vi "GoTo Tangent.vi"(7 "IA State Input in":T2, 8 "distance between ball and robot":dbl=250.0 format="%#_13g", 9 "Ball":dbl[](array[numeric])=[-1986.6092529296875, -3009.6396484375], 10 "Target":dbl[](array[numeric]), 11 "R":dbl[](array[numeric])=[-2840.578369140625, -1536.7857666015625, -1.0371381044387817]) -> (1 "Destination":dbl[](array[numeric]), 2 "Output\nVelocity":dbl[](array[numeric]) format="%.2f")   [LabVIEW 2016]
uses:
  Core/AI Input.ctl
  Core/AI Robot.ctl
  Intel/Functions Enum.ctl
  Intel/AttackerStates.ctl
  Core/AI Ball.ctl
  Core/Field Size.ctl
  Core/AI Judge.ctl
  Intel/Command Enum.ctl
  Util/Events/Events.ctl
  <vilib>/Analysis/coordinate.llb/Angle Range (Degree).ctl
  <vilib>/Analysis/coordinate.llb/Wrap Angle (scalar).vi
  <vilib>/Analysis/coordinate.llb/2D Cartesian Coordinate Rotation (Scalar).vi
  <vilib>/Analysis/NI_AALPro.lvlib
  <vilib>/Analysis/NI_AAL_Angle.lvlib
panel:
  in  "angle range":T1=1 items=["none", "-180 to 180 (-pi to pi)", "0 to 360 (0 to 2pi)"]
  out "Waveform Chart 2":dbl[][](graph)
  out "Robot":dbl[](array[numeric])=[-2840.578369140625, -1536.7857666015625, -1.0371381044387817]
  out "Waveform Chart":dbl[][](graph)
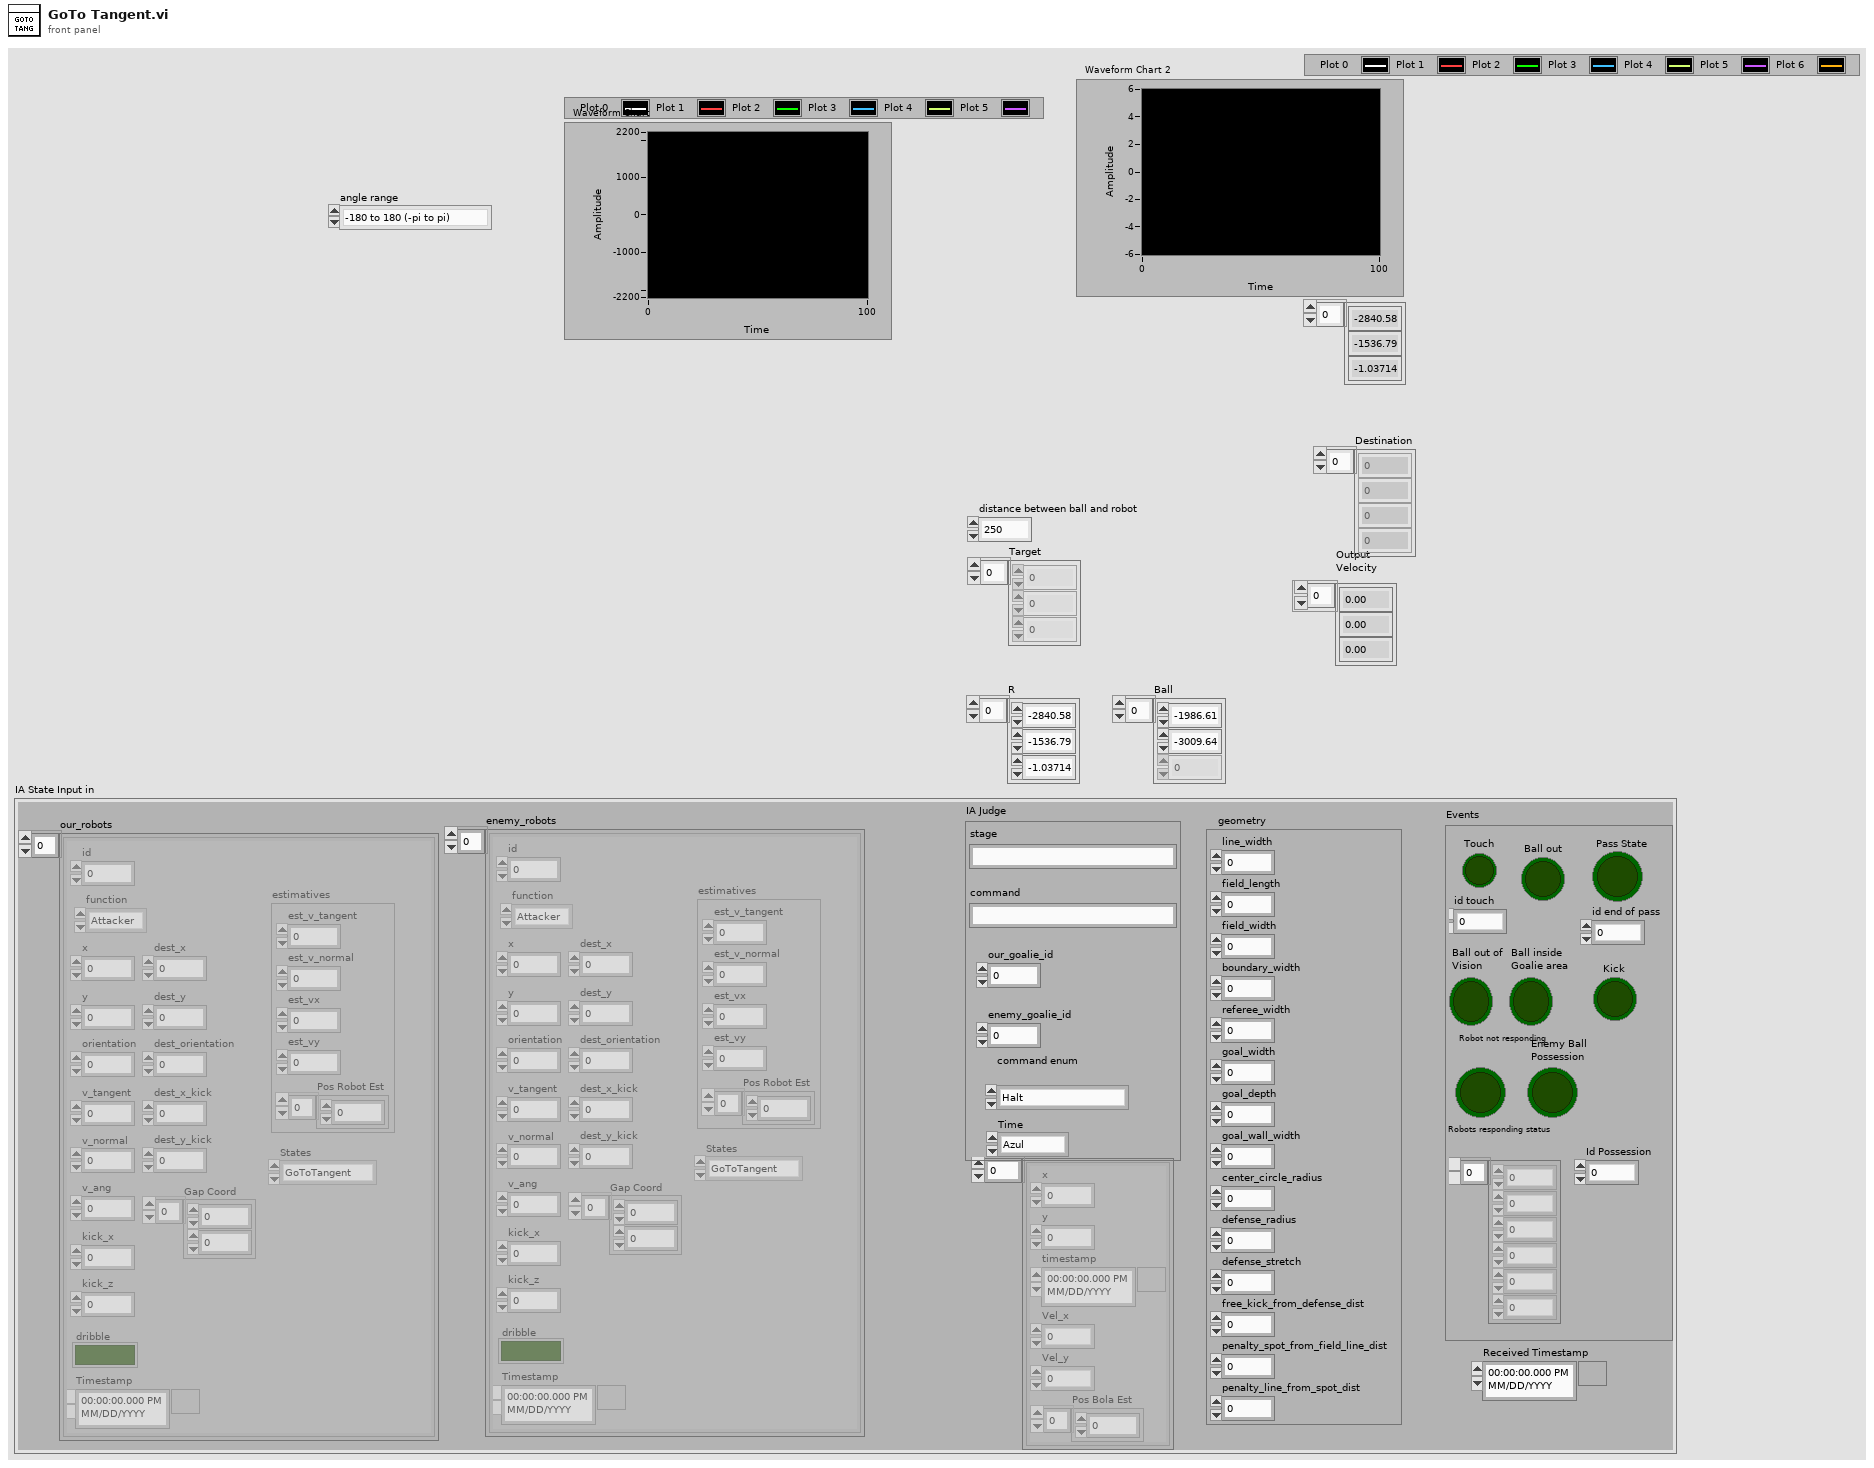
[diagram p1: front panel]
types:
  T1 = typedef "NI_AAL_Angle.lvlib/Angle Range (Degree).ctl" = u16
  T2 = typedef "AI Input.ctl" = cluster{"our_robots":T3[], "enemy_robots":T3[], "balls":T6[], "geometry":T7, "IA Judge":T8, "Received Timestamp":timestamp, "Events":T10}
  T3 = typedef "AI Robot.ctl" = cluster{"id":u32, "function":T4, "x":dbl, "y":dbl, "orientation":dbl, "v_tangent":dbl, "v_normal":dbl, "v_ang":dbl, "kick_x":dbl, "kick_z":dbl, "dribble":bool, "Timestamp":timestamp, "dest_x":dbl, "dest_y":dbl, "dest_orientation":dbl, "estimatives":cluster{"est_v_tangent":dbl, "est_v_normal":dbl, "est_vx":dbl, "est_vy":dbl, "Pos Robot Est":dbl[]}, "dest_x_kick":dbl, "dest_y_kick":dbl, "Gap Coord":dbl[], "States":T5}
  T4 = typedef "Functions Enum.ctl" = enum16{"Attacker", "Goalie", "Defender", "Striker", "Goto 0", "Dummy", "Kicker", "ZigZag"}
  T5 = typedef "AttackerStates.ctl" = enum16{"Pass", "GoToTangent", "BallGetting", "GoToKick", ""}
  T6 = typedef "AI Ball.ctl" = cluster{"x":dbl, "y":dbl, "timestamp":timestamp, "Vel_x":dbl, "Vel_y":dbl, "Pos Bola Est":dbl[]}
  T7 = typedef "Field Size.ctl" = cluster{"line_width":u32, "field_length":u32, "field_width":u32, "boundary_width":u32, "referee_width":u32, "goal_width":u32, "goal_depth":u32, "goal_wall_width":u32, "center_circle_radius":u32, "defense_radius":u32, "defense_stretch":u32, "free_kick_from_defense_dist":u32, "penalty_spot_from_field_line_dist":u32, "penalty_line_from_spot_dist":u32}
  T8 = typedef "AI Judge.ctl" = cluster{"stage":string, "command":string, "our_goalie_id":dbl, "enemy_goalie_id":dbl, "command enum":T9, "Time":enum16{"Azul", "Amarelo"}}
  T9 = typedef "Command Enum.ctl" = enum16{"Halt", "Stop", "Force Start", "PKA Normal Start", "Prepare Kickoff Ally", "PKE Normal Start", "Prepare Kickoff Enemy", "Prepare Penalty Ally", "PPA Normal Start", "Prepare Penalty Enemy", "PPE Normal Start", "Direct Free Enemy", "Direct Free Ally", "Indirect Free Enemy", "Indirect Free Ally", "Timeout Enemy", "Timeout Ally", "Goal Enemy", "Goal Ally", "Ball Placement Enemy", "Ball Placement Ally", "Normal Half Time", "Extra Time Break", "Extra Half Time", "None"}
  T10 = typedef "Events.ctl" = cluster{"Touch":bool, "Ball out":bool, "id touch":dbl, "Ball out of \nVision":bool, "Ball inside \nGoalie area":bool, "Robot not responding":bool, "Robots responding status":dbl[], "Enemy Ball \nPossession":bool, "Pass State":bool, "id end of pass":dbl, "Kick":bool, "Id Possession":dbl}
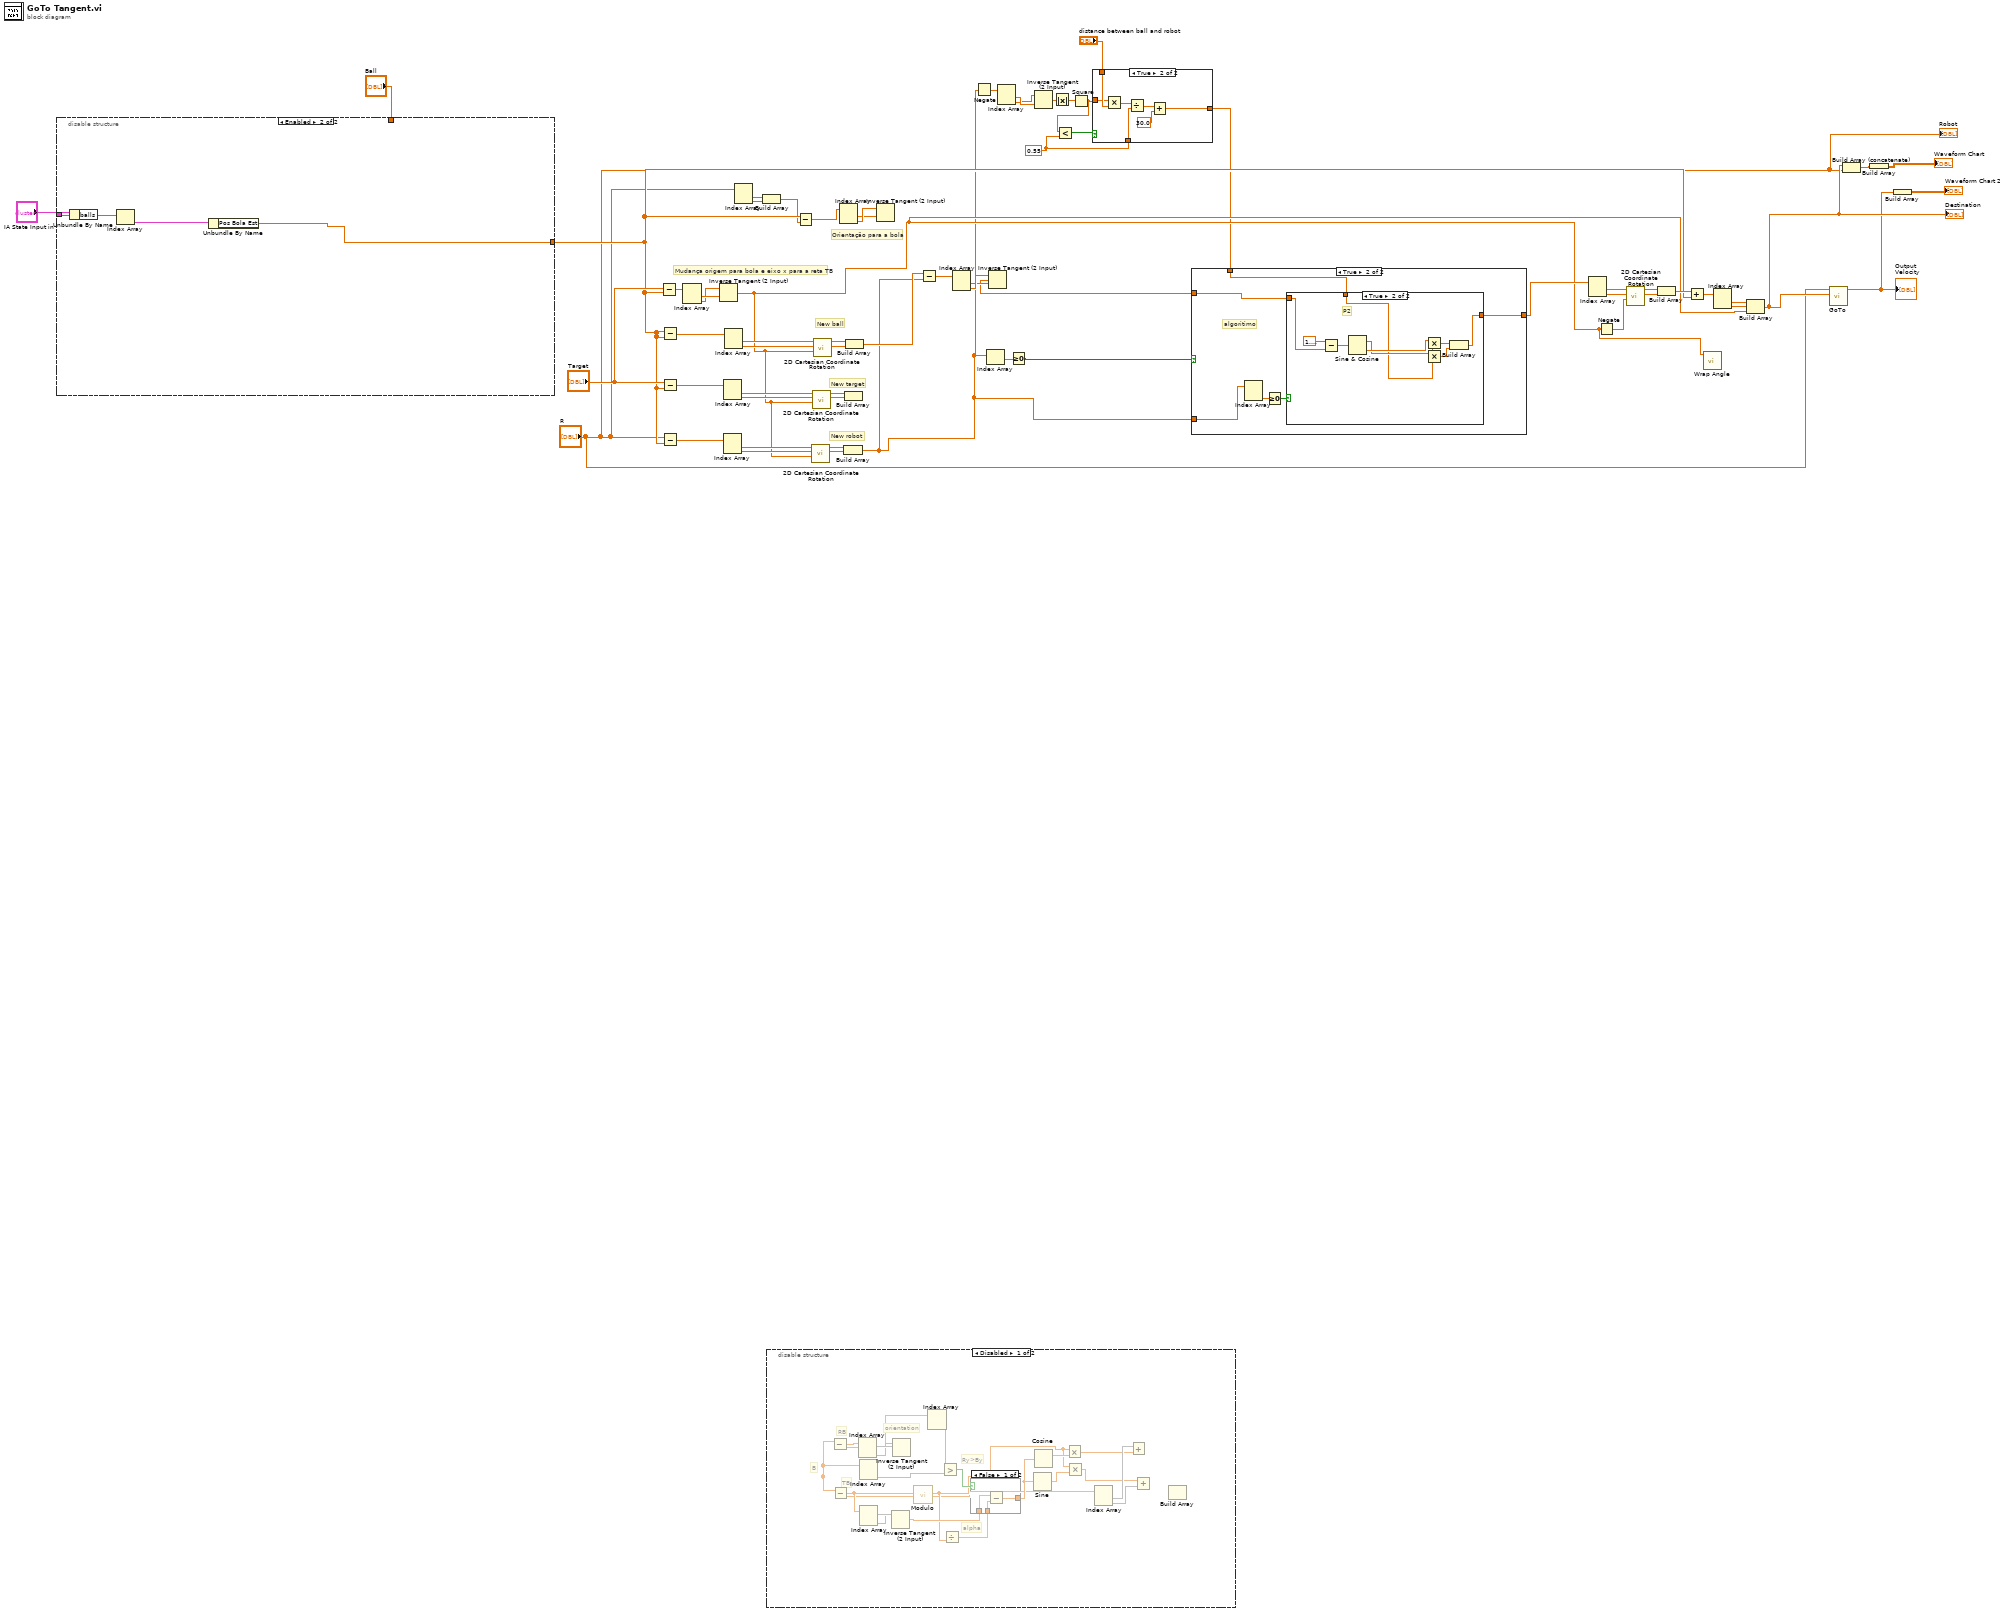
[diagram p0: block diagram]
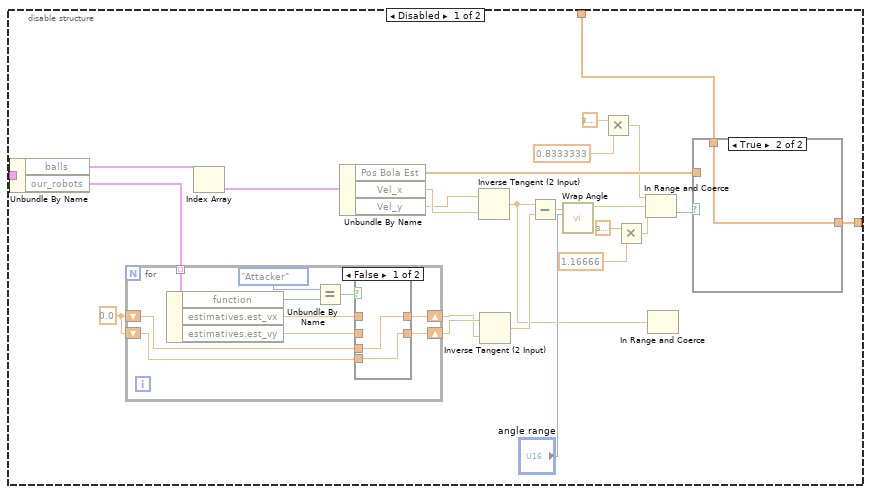
[diagram p3: hidden frame]
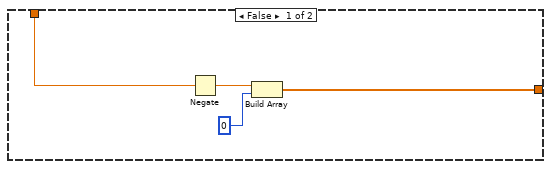
[diagram p6: hidden frame]
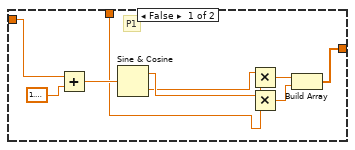
[diagram p7: hidden frame]
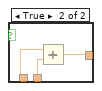
[diagram p8: hidden frame]
diagram:
  w5 = 0.55 ("y")
  # "New ball"
  # "New target"
  # "New robot"
  # "Orientação para a bola"
  # "Mudança origem para bola e eixo x para a reta TB"
  n1 = disable-structure shown="Enabled" {
    disable-tunnel: [w87 w103] -> w19
    disable-tunnel: "IA State Input in" -> [w86 w106]
    disable-tunnel: "Ball" -> [w64 _]
    frame Disabled {
      w82 = 0.0 ("est_vx")
      n2 = Unbundle By Name(w86) -> ("balls"=w85:T6[], "our_robots"=w83:T3[])
      n3 = for {
        tunnel: w83 -> [w97] mode=indexing
        shift-right: [w93] -> w79
        shift-left: w82 -> [w89]
        shift-right: [w90] -> w80
        shift-left: w82 -> [w88]
        n4 = Unbundle By Name(w97) -> ("function"=w95:T4, "estimatives.est_vx"=w92:dbl, "estimatives.est_vy"=w91:dbl)
        n5 = Equal?(x=Functions_Enum."Attacker" ("function"), y=w95) -> (x = y?=w96:bool)
        n6 = case shown="False" w96 {
          tunnel: [w99 w101] -> w93
          tunnel: w92 -> [_ w101]
          tunnel: w91 -> [_ w100]
          tunnel: [w98 w100] -> w90
          tunnel: w89 -> [w99 _]
          tunnel: w88 -> [w98 _]
          frame False {
          }
          frame True {
          }
        }
      }
      n7 = Index Array(array=w85) -> (element=w84:T6)  [unwired: 1 in]
      n8 = Unbundle By Name(w84) -> ("Pos Bola Est"=w81:dbl[], "Vel_x"=w78:dbl, "Vel_y"=w77:dbl)
      n9 = Inverse Tangent (2 Input)(1:w78, 2:w77) -> (0:w65:dbl)
      n10 = Inverse Tangent (2 Input)(1:w79, 2:w80) -> (0:w76:dbl)
      n11 = Subtract(x=w65, y=w76) -> (x-y=w74:dbl)
      n12 = call-poly <vilib>:"Wrap Angle.vi"("angle range"="angle range", "angle in"=w74) -> ("angle out"=w70:dbl)  [unwired: 8 in, 1 out]
      n13 = Multiply(x=3.141592653589793, y=0.8333333) -> (x*y=w67:dbl)
      n14 = Multiply(x=3.141592653589793, y=1.16666) -> (x*y=w73:dbl)
      n15 = In Range and Coerce(upper limit=w67, x=w70, lower limit=w73) -> (In Range?=w66:bool)  [unwired: 1 out]
      n16 = In Range and Coerce(x=w65) -> ()  [unwired: 2 in, 2 out]
      n17 = case shown="True" w66 {
        tunnel: [_ w102] -> w87
        tunnel: w81 -> [_ _]
        tunnel: w64 -> [_ w102]
        frame False {
        }
        frame True {
        }
      }
    }
    frame Enabled {
      n18 = Unbundle By Name(w106) -> ("balls"=w104:T6[])
      n19 = Index Array(array=w104) -> (element=w105:T6)  [unwired: 1 in]
      n20 = Unbundle By Name(w105) -> ("Pos Bola Est"=w103:dbl[])
    }
  }
  n21 = Subtract(x="Target", y=w19) -> (x-y=w54:dbl[])
  n22 = Subtract(x=w19, y=w19) -> (x-y=w61:dbl[])
  n23 = Subtract(x="Target", y=w19) -> (x-y=w58:dbl[])
  n24 = Subtract(x="R", y=w19) -> (x-y=w55:dbl[])
  n25 = Index Array(array=w54) -> (element #1=w53:dbl, element #2=w52:dbl)  [unwired: 2 in]
  n26 = Inverse Tangent (2 Input)(1:w53, 2:w52) -> (0:w12:dbl)
  n27 = Index Array(array=w55) -> (element #1=w57:dbl, element #2=w56:dbl)  [unwired: 2 in]
  n28 = Index Array(array=w58) -> (element #1=w60:dbl, element #2=w59:dbl)  [unwired: 2 in]
  n29 = Index Array(array=w61) -> (element #1=w63:dbl, element #2=w62:dbl)  [unwired: 2 in]
  n30 = Index Array(array="R") -> (element #1=w17:dbl, element #2=w16:dbl)  [unwired: 2 in]
  n31 = Build Array(w17, w16) -> (w15:dbl[])
  n32 = disable-structure shown="Disabled" {
    frame Disabled {
      # "Ry>By"
      # "orientation"
      # "RB"
      # "alpha"
      # "TB"
      # "B"
      n33 = Index Array() -> (array=w112:dbl[], element #2=w118)  [unwired: 2 in, 1 out]
      n34 = Index Array() -> (array=w108:dbl[], element #2=w119)  [unwired: 2 in, 1 out]
      n35 = Subtract(x=w112, y=w108) -> (x-y=w126:dbl)
      n36 = Index Array(array=w126) -> (element #1=w128, element #2=w127)  [unwired: 2 in]
      n37 = Inverse Tangent (2 Input)(1:w128, 2:w127) -> (0:w125:dbl)
      n38 = Greater?(x=w119, y=w118) -> (0:w117:bool)
      n39 = Index Array() -> (array=w107:dbl[], element #1=w115, element #2=w110)  [unwired: 2 in]
      n40 = Subtract(x=w112, y=w107) -> (x-y=w130:dbl)
      n41 = Index Array(array=w130) -> (element #1=w132, element #2=w131)  [unwired: 2 in]
      n42 = Inverse Tangent (2 Input)(1:w132, 2:w131) -> (0:w124:dbl)
      n43 = call "Modulo.vi"("2D vector"=w130) -> ("Modulo"=w116:dbl)  [unwired: 10 in]
      n44 = Divide(y=w116) -> (x=w129:dbl, x/y=w123:dbl)
      n45 = case shown="False" w117 {
        tunnel: w124 -> [w134 w138]
        tunnel: w123 -> [w135 w137]
        tunnel: [w133 w136] -> w122
        frame False {
          n46 = Subtract(x=w134, y=w135) -> (x-y=w133:dbl)
        }
        frame True {
          n47 = Add(x=w138, y=w137) -> (x+y=w136:dbl)
        }
      }
      n48 = Sine(x=w122) -> (sin(x)=w120:dbl)
      n49 = Cosine(x=w122) -> (cos(x)=w121:dbl)
      n50 = Multiply(x=w116, y=w121) -> (x*y=w114:dbl)
      n51 = Multiply(x=w116, y=w120) -> (x*y=w111:dbl)
      n52 = Add(x=w115, y=w114) -> (x+y=w113:dbl)
      n53 = Add(x=w111, y=w110) -> (x+y=w109:dbl)
      n54 = Build Array() -> ()  [unwired: 3 in, 1 out]
    }
    frame Enabled {
    }
  }
  n55 = Subtract(x=w19, y=w15) -> (x-y=w34:dbl[])
  n56 = call-poly <vilib>:"2D Cartesian Coordinate Rotation.vi"("theta"=w12, "y"=w56, "x"=w57) -> ("y out"=w46:dbl, "x out"=w47:dbl)  [unwired: 6 in, 1 out]
  n57 = call-poly <vilib>:"2D Cartesian Coordinate Rotation.vi"("theta"=w12, "y"=w59, "x"=w60) -> ("y out"=w50:dbl, "x out"=w51:dbl)  [unwired: 6 in, 1 out]
  n58 = call-poly <vilib>:"2D Cartesian Coordinate Rotation.vi"("theta"=w12, "y"=w62, "x"=w63) -> ("y out"=w48:dbl, "x out"=w49:dbl)  [unwired: 6 in, 1 out]
  n59 = Index Array(array=w34) -> (element #1=w35:dbl, element #2=w36:dbl)  [unwired: 2 in]
  n60 = Build Array(w47, w46) -> (w11:dbl[])
  n61 = Build Array(w51, w50) -> ()  [unwired: 1 out]
  n62 = Build Array(w49, w48) -> (w27:dbl[])
  n63 = Inverse Tangent (2 Input)(1:w35, 2:w36) -> ()  [unwired: 1 out]
  n64 = Subtract(x=w27, y=w11) -> (x-y=w43:dbl[])
  n65 = Index Array(array=w43) -> (element #1=w44:dbl, element #2=w45:dbl)  [unwired: 2 in]
  n66 = Negate(x=w11) -> (-x=w10:dbl[])
  n67 = Index Array(array=w11) -> (element=w29:dbl)  [unwired: 1 in]
  n68 = Inverse Tangent (2 Input)(1:w44, 2:w45) -> (0:w28:dbl)
  n69 = Index Array(array=w10) -> (element #1=w9:dbl, element #2=w8:dbl)  [unwired: 2 in]
  n70 = Greater Or Equal To 0?(x=w29) -> (x >= 0?=w30:bool)
  n71 = Inverse Tangent (2 Input)(1:w9, 2:w8) -> (0:w7:dbl)
  n72 = Absolute Value(x=w7) -> (abs(x)=w2:dbl)
  n73 = Square(x=w2) -> (x^2=w1:dbl)
  n74 = Less?(x=w1, y=w5) -> (x < y?=w6:bool)
  n75 = case shown="True" w6 {
    tunnel: w5 -> [_ w143]
    tunnel: [w139 w142] -> w4
    tunnel: "distance between ball and robot" -> [w139 w141]
    tunnel: w1 -> [_ w140]
    frame False {
    }
    frame True {
      n76 = Multiply(x=w140, y=w141) -> (x*y=w146:dbl)
      n77 = Divide(x=w146, y=w143) -> (x/y=w145:dbl)
      n78 = Add(x=w145, y=30.0) -> (x+y=w142:dbl)
    }
  }
  n79 = case shown="True" w30 {
    tunnel: w28 -> [_ w155]
    tunnel: [w149 w154] -> w38
    tunnel: w11 -> [_ w152]
    tunnel: w4 -> [w147 w151]
    frame False {
      n80 = Negate(x=w147) -> (-x=w148:dbl)
      n81 = Build Array(w148, 0 ("index")) -> (w149:dbl[])
    }
    frame True {
      # "algoritimo"
      n82 = Index Array(array=w152) -> (element #2=w156:dbl)  [unwired: 2 in, 1 out]
      n83 = Greater Or Equal To 0?(x=w156) -> (x >= 0?=w153:bool)
      n84 = case shown="True" w153 {
        tunnel: w155 -> [w159 w167]
        tunnel: [w161 w170] -> w154
        tunnel: w151 -> [w157 w166]
        frame False {
          # "P1"
          n85 = Add(x=w159, y=1.5707963267948966) -> (x+y=w160:dbl)
          n86 = Sine & Cosine(0:w160) -> (1:w163:dbl, 2:w162:dbl)
          n87 = Multiply(x=w162, y=w157) -> (x*y=w165:dbl)
          n88 = Multiply(x=w163, y=w157) -> (x*y=w164:dbl)
          n89 = Build Array(w165, w164) -> (w161:dbl[])
        }
        frame True {
          # "P2"
          n90 = Subtract(x=1.5707963267948966, y=w167) -> (x-y=w169:dbl)
          n91 = Sine & Cosine(0:w169) -> (1:w173:dbl, 2:w174:dbl)
          n92 = Multiply(x=w174, y=w166) -> (x*y=w171:dbl)
          n93 = Multiply(x=w173, y=w166) -> (x*y=w172:dbl)
          n94 = Build Array(w171, w172) -> (w170:dbl[])
        }
      }
    }
  }
  n95 = Index Array(array=w38) -> (element #1=w42:dbl, element #2=w41:dbl)  [unwired: 2 in]
  n96 = Negate(x=w12) -> (-x=w24:dbl)
  n97 = call-poly <vilib>:"2D Cartesian Coordinate Rotation.vi"("theta"=w24, "y"=w41, "x"=w42) -> ("y out"=w39:dbl, "x out"=w40:dbl)  [unwired: 6 in, 1 out]
  n98 = Build Array(w40, w39) -> (w37:dbl[])
  n99 = Add(x=w37, y=w19) -> (x+y=w33:dbl[])
  n100 = call-poly <vilib>:"Wrap Angle.vi"("angle in"=w12) -> ()  [unwired: 9 in, 2 out]
  n101 = Index Array(array=w33) -> (element #1=w32:dbl, element #2=w31:dbl)  [unwired: 2 in]
  n102 = Build Array(w32, w31, w12) -> (w26:dbl[])
  "Destination" <- w26
  n103 = call "GoTo.vi"("Target"=w26, "Position"="R") -> ("Output\nVelocity"=w25:dbl[])  [unwired: 8 in, 1 out]
  "Output\nVelocity" <- w25
  n104 = Build Array (concatenate)(w26, "R") -> (w23:dbl[])
  n105 = Build Array(w23) -> (→"Waveform Chart":dbl[][])
  n106 = Build Array(w25) -> (→"Waveform Chart 2":dbl[][])
  "Robot" <- "R"
